vi "Filter Events.vi"(4 "Events":T2[](array[typedef]), 5 "Event Filters":T1) -> (7 "Filtered Events":T2[](array[typedef]))   [LabVIEW 2020, in "VolatusGUI.lvlib" / "Event Viewer Module.lvclass"]
uses:
  Event Viewer Module.lvclass
  Event Element.ctl
  Event Filters.ctl
  Event Viewer Module.lvclass/Event Viewer Module.ctl
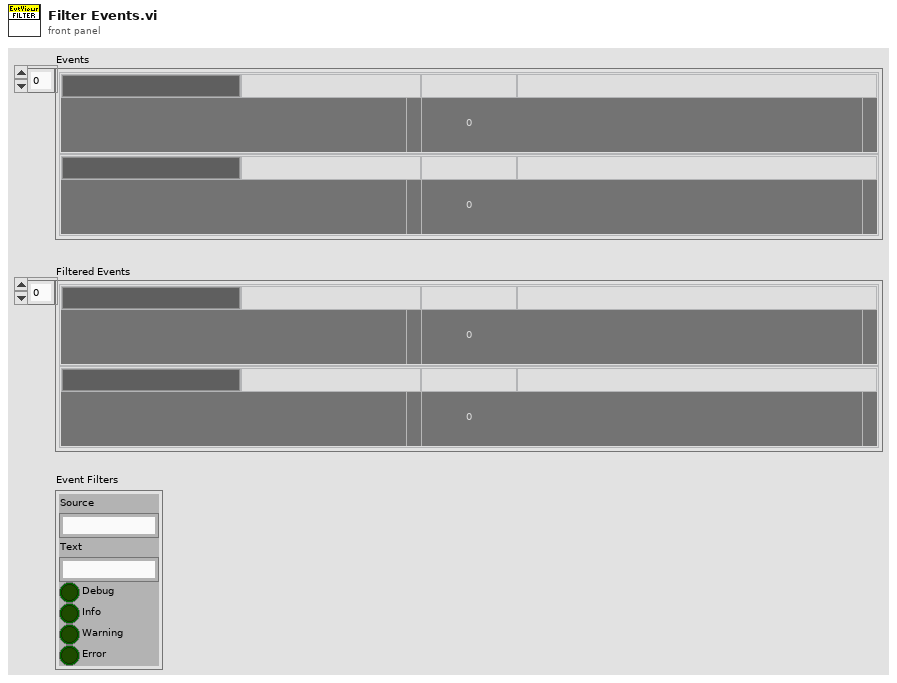
[diagram p1: front panel]
types:
  T1 = typedef "VolatusGUI.lvlib/Event Viewer Module.lvclass/Event Filters.ctl" = cluster{"Source":string, "Text":string, "Debug":bool, "Info":bool, "Warning":bool, "Error":bool}
  T2 = typedef "VolatusGUI.lvlib/Event Viewer Module.lvclass/Event Element.ctl" = cluster{"Node":string, "Node Color":u32, "Timestamp":string, "TS Color":u32, "Level":string, "Level Color":u32, "Context":string, "Context Color":u32, "Message":string, "Error Code":i32, "Error Source":string}
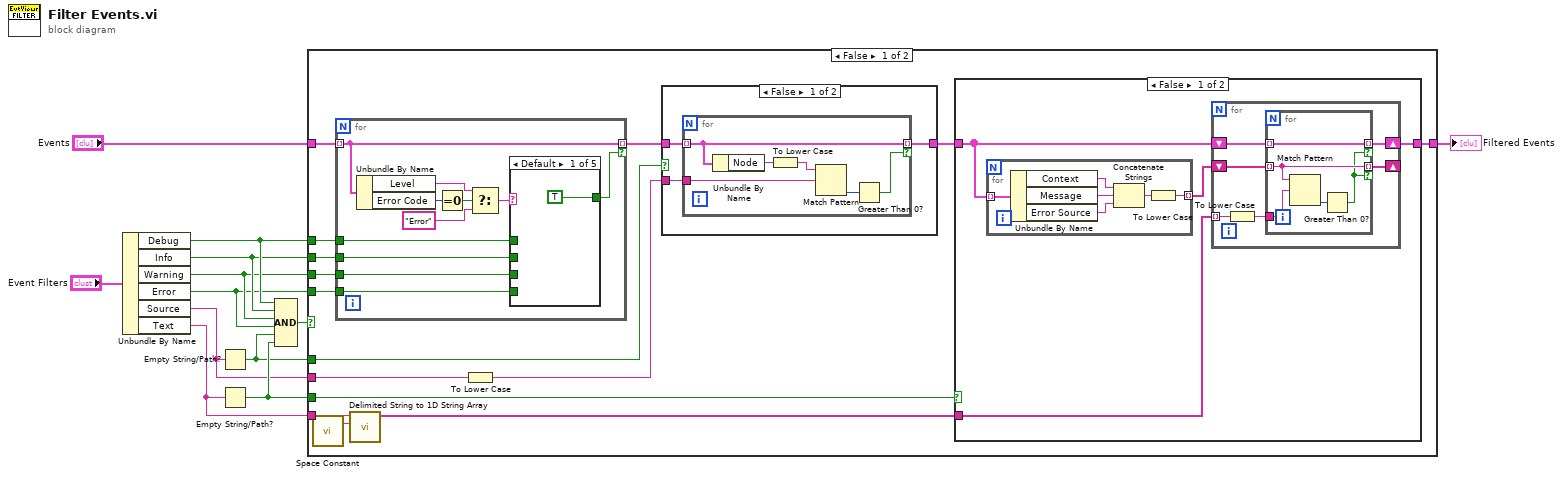
[diagram p0: block diagram]
diagram:
  n1 = Unbundle By Name("Event Filters") -> ("Debug"=w10:bool, "Info"=w9:bool, "Warning"=w8:bool, "Error"=w7:bool, "Source"=w2:string, "Text"=w3:string)
  n2 = Empty String/Path?(string/path=w2) -> (empty?=w1:bool)
  n3 = Empty String/Path?(string/path=w3) -> (empty?=w11:bool)
  n4 = Compound Arithmetic op=AND(w10, w9, w8, w7, w1, w11) -> (w12:bool)
  n5 = case shown="False" w12 {
    tunnel: w7 -> [w23 _]
    tunnel: w8 -> [w24 _]
    tunnel: w9 -> [w25 _]
    tunnel: w10 -> [w26 _]
    tunnel: w3 -> [w20 _]
    tunnel: [w21 w76] -> w6
    tunnel: "Events" -> [w27 w76]
    tunnel: w11 -> [w22 _]
    tunnel: w2 -> [w15 _]
    tunnel: w1 -> [w16 _]
    frame False {
      n6 = call <vilib>:"Space Constant.vi"() -> ("String"=w19:string)
      n7 = for {
        tunnel: w27 -> [w39] mode=indexing
        tunnel: w26 -> [w43]
        tunnel: w25 -> [w42]
        tunnel: w24 -> [w41]
        tunnel: w23 -> [w40]
        tunnel: [w39] -> w17 mode=indexing if=w38
        n8 = Unbundle By Name(w39) -> ("Level"=w46:string, "Error Code"=w48:i32)
        n9 = Equal To 0?(x=w48) -> (x = 0?=w47:bool)
        n10 = Select(t=w46, s=w47, f="Error") -> (s? t:f=w44:string)
        n11 = case shown="Default" w44 {
          tunnel: w43 -> [_ w50 _ _ _]
          tunnel: w42 -> [_ _ w51 _ _]
          tunnel: w41 -> [_ _ _ w52 _]
          tunnel: w40 -> [_ _ _ _ w53]
          tunnel: [TRUE ("Error") w50 w51 w52 w53] -> w38
          frame Default {
          }
          frame "Debug" {
          }
          frame "Info" {
          }
          frame "Warning" {
          }
          frame "Error" {
          }
        }
      }
      n12 = call <vilib>:"Delimited String to 1D String Array.vi"("delimiter"=w19, "delimited string"=w20) -> ("string array"=w18:string[])  [unwired: 9 in]
      n13 = To Lower Case(string=w15) -> (all lower case string=w13:string)
      n14 = case shown="False" w16 {
        tunnel: w17 -> [w30 w37]
        tunnel: w13 -> [w28 _]
        tunnel: [w29 w37] -> w14
        frame False {
          n15 = for {
            tunnel: w30 -> [w36] mode=indexing
            tunnel: [w36] -> w29 mode=indexing if=w32
            tunnel: w28 -> [w34]
            n16 = Unbundle By Name(w36) -> ("Node"=w35:string)
            n17 = To Lower Case(string=w35) -> (all lower case string=w31:string)
            n18 = Match Pattern(string=w31, regular expression=w34) -> (offset past match=w33:i32)  [unwired: 1 in, 3 out]
            n19 = Greater Than 0?(x=w33) -> (x > 0?=w32:bool)
          }
        }
        frame True {
        }
      }
      n20 = case shown="False" w22 {
        tunnel: [w55 w75] -> w21
        tunnel: w14 -> [w56 w75]
        tunnel: w18 -> [w54 _]
        frame False {
          n21 = for {
            tunnel: w56 -> [w74] mode=indexing
            tunnel: [w69] -> w57 mode=indexing
            n22 = Unbundle By Name(w74) -> ("Context"=w73:string, "Message"=w72:string, "Error Source"=w71:string)
            n23 = Concatenate Strings(w73, w72, w71) -> (w70:string)
            n24 = To Lower Case(string=w70) -> (all lower case string=w69:string)
          }
          n25 = for {
            shift-right: [w60] -> _
            shift-left: w57 -> [w62]
            shift-right: [w61] -> w55
            shift-left: w56 -> [w63]
            tunnel: w54 -> [w59] mode=indexing
            n26 = To Lower Case(string=w59) -> (all lower case string=w58:string)
            n27 = for {
              tunnel: w63 -> [w68] mode=indexing
              tunnel: w62 -> [w66] mode=indexing
              tunnel: [w68] -> w61 mode=indexing if=w64
              tunnel: [w66] -> w60 mode=indexing if=w64
              tunnel: w58 -> [w67]
              n28 = Match Pattern(string=w66, regular expression=w67) -> (offset past match=w65:i32)  [unwired: 1 in, 3 out]
              n29 = Greater Than 0?(x=w65) -> (x > 0?=w64:bool)
            }
          }
        }
        frame True {
        }
      }
    }
    frame True {
      # "No filtering"
    }
  }
  "Filtered Events" <- w6
